vi "SetIndividualJoints.vi"(0 "Mode":T1=1 items=["Position"=1, "Velocity"=2, "Effort"=3], 1 "node":string, 2 "Joint States":T2(array[cluster]), 3 "error in":errorcluster) -> (6 "error out":errorcluster)   [LabVIEW 2010]
uses:
  ROS/Code/SubVIs/BaxterSide.ctl
  ROS/Code/SubVIs/_ROSDirection.ctl
  ROS/Code/Console/Servers/ServerSubs/TopicDef.ctl
  ROS/MessageBuilding/std_msgs/subs/i32Scalar.vi
  ROS/Code/SubVIs/JointMode.ctl
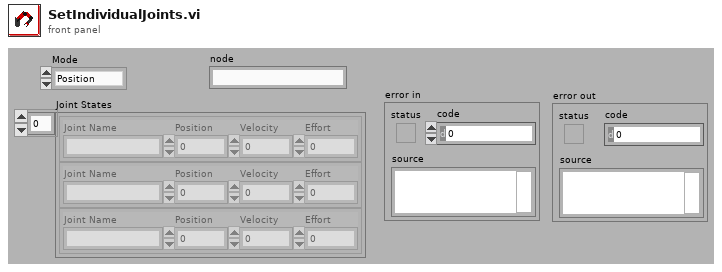
[diagram p1: front panel]
types:
  T1 = typedef "JointMode.ctl" = u8
  T2 = cluster{"Joint Name":string, "Position":dbl, "Velocity":dbl, "Effort":dbl}[]
  T3 = typedef "TopicDef.ctl" = cluster{"Topic":string, "Type":string, "Action":T4, "Update (ms)":u16, "write queue":u16}
  T4 = typedef "_ROSDirection.ctl" = enum16{"Node", "Publisher", "Subscriber", "Service Client"}
  T5 = typedef "BaxterSide.ctl" = enum16{"left", "right"}
  T6 = typedef "_ROSControl.ctl" = cluster{"topic port":u16, "Node":string, "topic":string, "type":string, "node port":u32, "error ":errorcluster, "Direction":T4, "APIs":string[], "Update (ms)":u16, "write queue":u16}
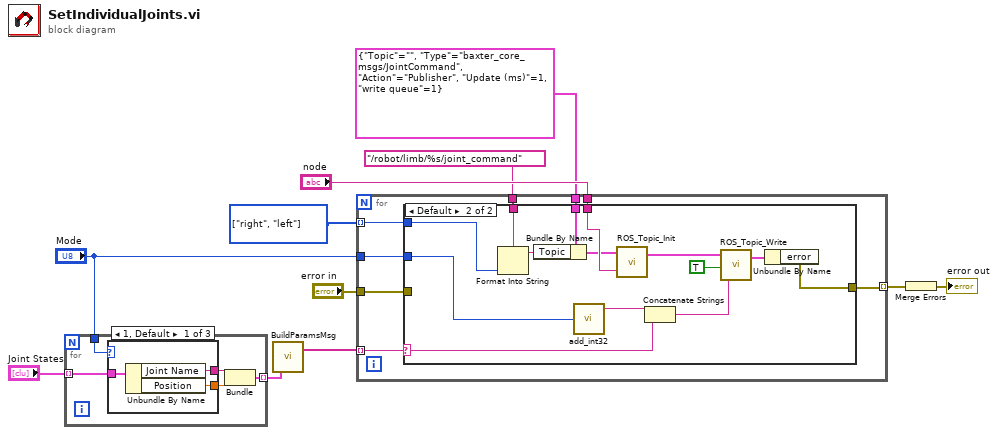
[diagram p0: block diagram]
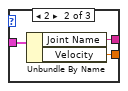
[diagram p2: hidden frame]
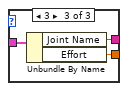
[diagram p3: hidden frame]
diagram:
  w9 = T5[] [enum."right", enum."left"] items=["left", "right"]
  n1 = for {
    tunnel: "Joint States" -> [w16] mode=indexing
    tunnel: "Mode" -> [w15]
    tunnel: [w12] -> w3 mode=indexing
    n2 = case shown="1, Default" w15 {
      tunnel: w16 -> [w19 w22 w25]
      tunnel: [w18 w21 w24] -> w14
      tunnel: [w17 w20 w23] -> w13
      frame 1, Default {
        n3 = Unbundle By Name(w19) -> ("Joint Name"=w18:string, "Position"=w17:dbl)
      }
      frame 2 {
        n4 = Unbundle By Name(w22) -> ("Joint Name"=w21:string, "Velocity"=w20:dbl)
      }
      frame 3 {
        n5 = Unbundle By Name(w25) -> ("Joint Name"=w24:string, "Effort"=w23:dbl)
      }
    }
    n6 = Bundle("Joint Name"=w14, "Effort"=w13) -> (w12:cluster{"Joint Name":string, "Effort":dbl})  [unwired: 1 in]
  }
  n7 = call "BuildParamsMsg.vi"("Parameters"=w3) -> ("Commands"=w1:string[])  [unwired: 1 in]
  n8 = for {
    tunnel: [w33] -> w7 mode=indexing
    tunnel: "error in" -> [w32]
    tunnel: "node" -> [w30]
    tunnel: w9 -> [w31] mode=indexing
    tunnel: "Mode" -> [w29]
    tunnel: w1 -> [w28] mode=indexing
    tunnel: "/robot/limb/%s/joint_command" ("topic") -> [w27]
    tunnel: T3 {"Topic"="", "Type"="baxter_core_msgs/JointCommand", "Action"=enum."Publisher", "Update (ms)"=1, "write queue"=1} ("Definitions") -> [w26]
    n9 = case shown="Default" w28 {
      selector: w28 -> [_ w37]
      tunnel: [w34 w40] -> w33
      tunnel: w32 -> [w34 _]
      tunnel: w31 -> [_ w47]
      tunnel: w30 -> [_ w46]
      tunnel: w29 -> [_ w39]
      tunnel: w27 -> [_ w45]
      tunnel: w26 -> [_ w43]
      frame "" {
      }
      frame Default {
        n10 = Format Into String(format string=w45, w47) -> (resulting string=w44:string)  [unwired: 2 in, 1 out]
        n11 = Bundle By Name(cluster=w43, "Topic"=w44) -> (w42:T3)
        n12 = call-poly "add_int32.vi"("Numeric"=w39) -> ("msg out"=w38:string)  [unwired: 4 in]
        n13 = call "ROS_Topic_Init.vi"("node"=w46, "Definitions"=w42) -> ("ROS out"=w48:T6)  [unwired: 1 in]
        n14 = Concatenate Strings(w38, w37) -> (w36:string)
        n15 = call "ROS_Topic_Write.vi"("Msg in"=w36, "Continuous?"=TRUE, "ROS in"=w48) -> ("ROS out"=w41:T6)  [unwired: 1 in]
        n16 = Unbundle By Name(w41) -> ("error"=w40:errorcluster)
      }
    }
  }
  n17 = Merge Errors(w7) -> (→"error out":errorcluster)
